vi "exercice4-5.vi"() -> ()   [LabVIEW 2013]
panel:
  out "Historique  Temperature":cluster{"temeperature":dbl, dbl}(graph)
  in  "Stop":bool=TRUE
  # "Marche"
  # "Arret"
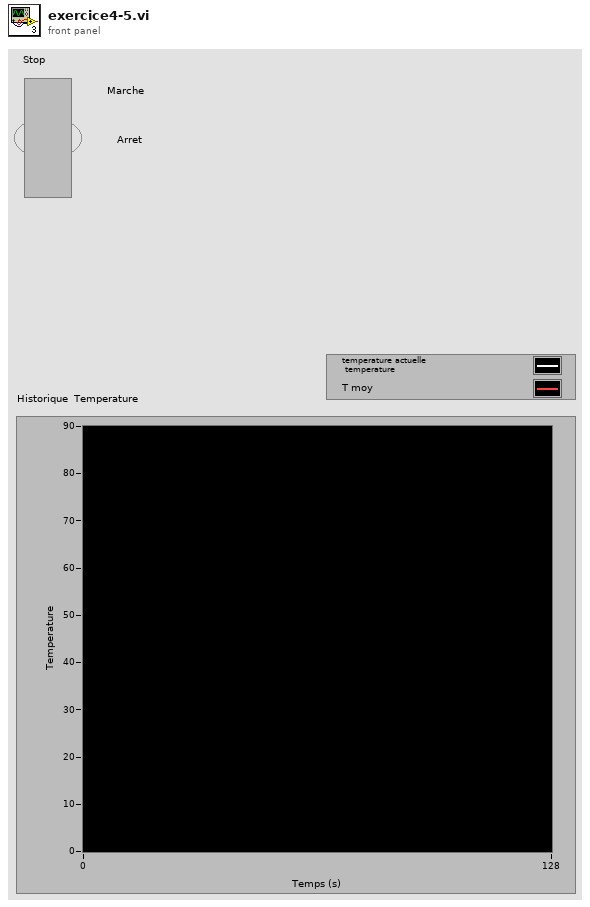
[diagram p1: front panel]
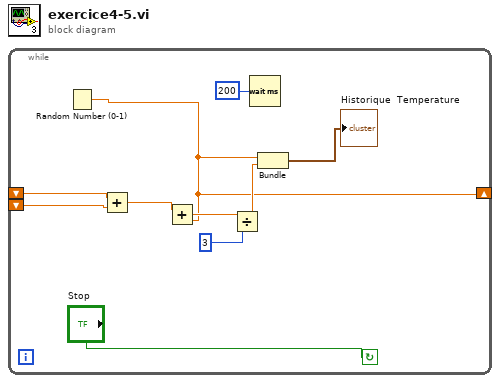
[diagram p0: block diagram]
diagram:
  n1 = while {
    shift-right: [w1] -> _
    shift-left: _ -> [w5]
    shift-left: _ -> [w4]
    stop <- "Stop" continue-if-true
    n2 = Random Number (0-1)() -> (number: 0 to 1=w1:dbl)
    n3 = Add(x=w5, y=w4) -> (x+y=w10:dbl)
    n4 = Add(x=w10, y=w1) -> (x+y=w9:dbl)
    n5 = Divide(x=w9, y=3) -> (x/y=w3:dbl)
    n6 = Wait (ms)(milliseconds to wait=200) -> ()  [unwired: 1 out]
    n7 = Bundle("number: 0 to 1"=w1, w3) -> (→"Historique  Temperature":cluster{"number: 0 to 1":dbl, dbl})  [unwired: 1 in]
  }
